vi "Generate UUID.vi"() -> (3 "UUID":string)   [LabVIEW 2017]
doc: "Generates a universally unique identifier and returns it as the standard 36-character UUID string."
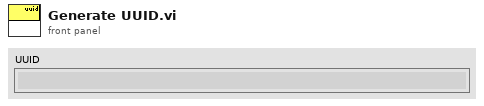
[diagram p1: front panel]
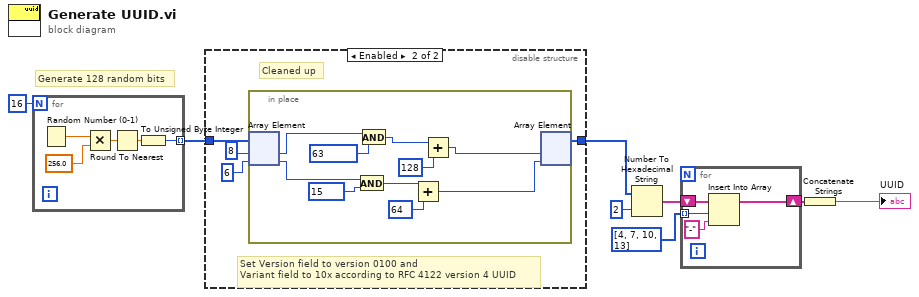
[diagram p0: block diagram]
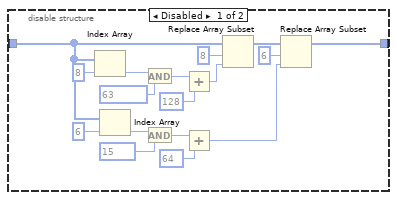
[diagram p2: hidden frame]
diagram:
  # "Generate 128 random bits"
  n1 = for {
    N: 16 -> [_]
    tunnel: [w9] -> w5 mode=indexing
    n2 = Random Number (0-1)() -> (number: 0 to 1=w13:dbl)
    n3 = Multiply(x=w13, y=256.0) -> (x*y=w11:dbl)
    n4 = Round To Nearest(number=w11) -> (nearest integer value=w10:dbl)
    n5 = To Unsigned Byte Integer(number=w10) -> (unsigned 8bit integer=w9:u8)
  }
  n6 = disable-structure shown="Enabled" {
    disable-tunnel: [w30 w33] -> w7
    disable-tunnel: w5 -> [w16 w34]
    frame Disabled {
      n7 = Index Array(array=w16, index=8) -> (element=w14:u8)
      n8 = Index Array(array=w16, index=6) -> (element=w17:u8)
      n9 = And(x=w14, y=u8 63) -> (x .and. y?=w21:u8)
      n10 = And(x=w17, y=u8 15) -> (x .and. y?=w24:u8)
      n11 = Add(x=w21, y=u8 128) -> (x+y=w20:u8)
      n12 = Add(x=w24, y=u8 64) -> (x+y=w22:u8)
      n13 = Replace Array Subset(array=w16, new element=w20, index=8) -> (w27:u8[])
      n14 = Replace Array Subset(array=w27, new element=w22, index=6) -> (w30:u8[])
    }
    frame Enabled {
      # "Cleaned up"
      # "Set Version field to version 0100 and \nVariant field to 10x according to RFC 4122 version 4 UUID"
      n15 = in-place {
        n16 = in-place-array #1(w34, 8 ("index"), 6 ("index")) -> (w43:u8, w42:u8)
        n17 = And(x=w42, y=u8 15) -> (x .and. y?=w39:u8)
        n18 = And(x=w43, y=u8 63) -> (x .and. y?=w37:u8)
        n19 = Add(x=w39, y=u8 64) -> (x+y=w35:u8)
        n20 = Add(x=w37, y=u8 128) -> (x+y=w36:u8)
        n21 = in-place-array #1(w36, w35) -> (w33:u8[])  [unwired: 2 out]
      }
    }
  }
  n22 = Number To Hexadecimal String(1:i16 2 ("width (-)"), 2:w7) -> (0:w3:string[])
  n23 = for {
    shift-right: [w47] -> w2
    shift-left: w3 -> [w48]
    tunnel: i32[] [4, 7, 10, 13] ("Array") -> [w45] mode=indexing
    n24 = Insert Into Array(array=w48, index=w45, new element="-" ("new element/subarray")) -> (w47:string[])
  }
  n25 = Concatenate Strings(w2) -> (→"UUID":string)
